vi "Execute Command.vi"(8 "error in (no error)":errorcluster, 10 "Robot Actors.lvlib:Command.lvlib:Command.lvclass":refnum<class "Command.lvclass">, 11 "Command Processor in":refnum<class "Command Processor.lvclass">) -> (0 "error out":errorcluster, 3 "Command Processor out":refnum<class "Command Processor.lvclass">)   [LabVIEW 2013]
uses:
  <vilib>/ActorFramework/Stop Msg/Stop Msg.lvclass
  <vilib>/ActorFramework/Actor/Actor.lvclass
  Command Processor.lvclass
  Command/Command Class/Command.lvclass
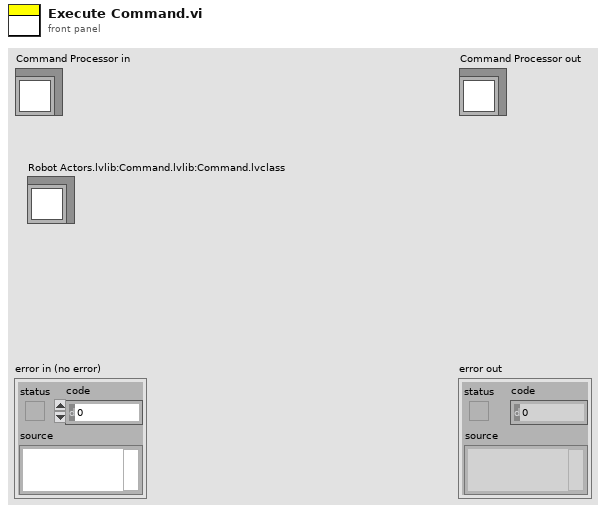
[diagram p1: front panel]
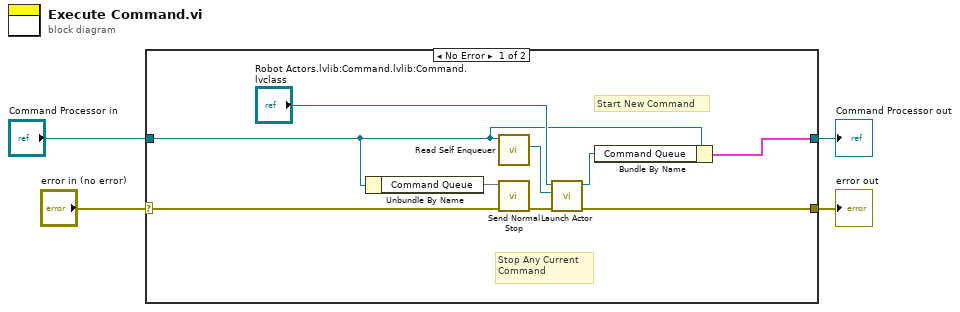
[diagram p0: block diagram]
diagram:
  n1 = case shown="No Error" "error in (no error)" {
    selector: "error in (no error)" -> [w8 w15]
    tunnel: [w7 w15] -> w3
    tunnel: [w12 w14] -> w1
    tunnel: "Command Processor in" -> [w6 w14]
    frame No Error {
      # "Start New Command"
      # "Stop Any Current \nCommand"
      n2 = Unbundle By Name(w6) -> ("Command Queue"=w13)
      n3 = call <vilib>:"Read Self Enqueuer.vi"("Actor"=w6) -> ("Self Enqueuer"=w5:refnum<class "Message Enqueuer.lvclass">)  [unwired: 10 in]
      n4 = call <vilib>:"Send Normal Stop.vi"("error in (no error)"=w8, "Message Enqueuer"=w13) -> ("error out"=w9:errorcluster)  [unwired: 9 in]
      n5 = call <vilib>:"Launch Actor.vi"("error in (no error)"=w9, "Actor-to-Caller Enqueuer"=w5, "Actor"="Robot Actors.lvlib:Command.lvlib:Command.lvclass") -> ("error out"=w7:errorcluster, "Caller-To-Actor Enqueuer"=w10:refnum<class "Message Enqueuer.lvclass">)  [unwired: 7 in]
      n6 = Bundle By Name(cluster=w6, "Command Queue"=w10) -> (w12:cluster{})
    }
    frame Error {
    }
  }
  "error out" <- w3
  "Command Processor out" <- w1
